vi "Template - Function Generator Arbitrary Waveform.vi"() -> ()   [LabVIEW 2020]
doc: "This example shows how to create then configure an arbitrary waveform."
uses:
  Instance           1 56Saved   Template - Function Generator Arbitrary Waveform .vi
  Instance           2 56Saved   Template - Function Generator Arbitrary Waveform .vi
  <instrlib>/_Template - Function Generator/Template - Function Generator.lvlib
panel:
  in  "Offset (0.00 V)":dbl
  in  "Frequency (1000 Hz)":dbl=1000.0
  in  "Gain (1.0)":dbl=1.0
  in  "Arbitrary Waveform Name":string="ARB1"
  in  "VISA resource name":refnum<visa-resource-name>
  # "(c) 2014 <Enter Company Name Here>.  ALL RIGHTS RESERVED."
  # "To edit the Arbitrary Waveform, use the Simulate Arbitrary Signal on the block diagram."
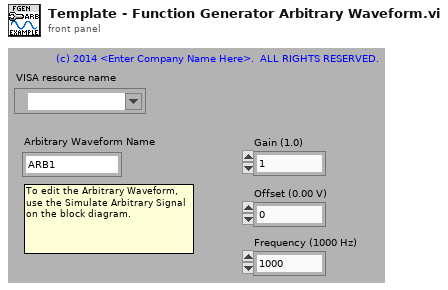
[diagram p1: front panel]
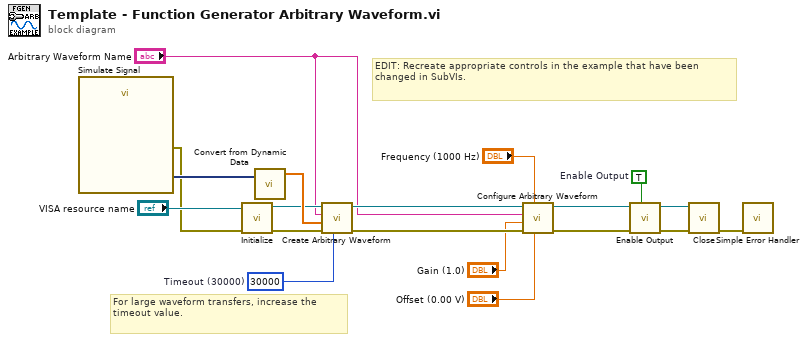
[diagram p0: block diagram]
diagram:
  w3 = TRUE  # Enable Output
  w13 = u32 30000  # Timeout (30000)
  # "EDIT: Recreate appropriate controls in the example that have been changed in SubVIs."
  # "For large waveform transfers, increase the timeout value."
  n1 = call "Simulate Signal"() -> ("Sine with Uniform Noise"=w19:dynamicdata, "error out"=w17:errorcluster)  [unwired: 14 in]
  n2 = call <instrlib>:"Initialize.vi"("error in (no error)"=w17, "VISA resource name"="VISA resource name") -> ("error out"=w12:errorcluster, "VISA resource name out"=w10:refnum<visa-resource-name>)  [unwired: 8 in]
  n3 = call "Convert from Dynamic Data"("Dynamic Data Type"=w19) -> ("Array"=w11:dbl[])  [unwired: 3 in]
  n4 = call <instrlib>:"Create Arbitrary Waveform.vi"("Timeout (10000 ms)"=w13, "error in (no error)"=w12, "Arbitrary Waveform Data"=w11, "Arbitrary Waveform Name (\"ARB1\")"="Arbitrary Waveform Name", "VISA resource name"=w10) -> ("error out"=w6:errorcluster, "VISA resource name out"=w9:refnum<visa-resource-name>)  [unwired: 5 in]
  n5 = call <instrlib>:"Configure Arbitrary Waveform.vi"("Offset (0.00 V)"="Offset (0.00 V)", "Frequency (1000 Hz)"="Frequency (1000 Hz)", "error in (no error)"=w6, "Gain (1.0 Vpp)"="Gain (1.0)", "Arbitrary Waveform Name (\"ARB1\")"="Arbitrary Waveform Name", "VISA resource name"=w9) -> ("error out"=w7:errorcluster, "VISA resource name out"=w8:refnum<visa-resource-name>)  [unwired: 4 in]
  n6 = call <instrlib>:"Enable Output.vi"("Enable Output (T: Enable)"=w3, "error in (no error)"=w7, "VISA resource name"=w8) -> ("error out"=w15:errorcluster, "VISA resource name out"=w14:refnum<visa-resource-name>)  [unwired: 7 in]
  n7 = call <instrlib>:"Close.vi"("error in (no error)"=w15, "VISA resource name"=w14) -> ("error out"=w16:errorcluster)  [unwired: 9 in]
  n8 = call <vilib>:"Simple Error Handler.vi"("error in (no error)"=w16) -> ()  [unwired: 4 in, 5 out]
